vi "Card Inserted.vi"(8 "error in (no error)":errorcluster, 11 "ATM Controller in":refnum<class "ATM Controller.lvclass">) -> (0 "error out":errorcluster, 3 "ATM Controller out":refnum<class "ATM Controller.lvclass">)   [LabVIEW 2020, in "ATM Controller.lvclass"]
uses:
  ATM Controller.lvclass
  State.ctl
  ATM Controller.lvclass/ATM Controller.ctl
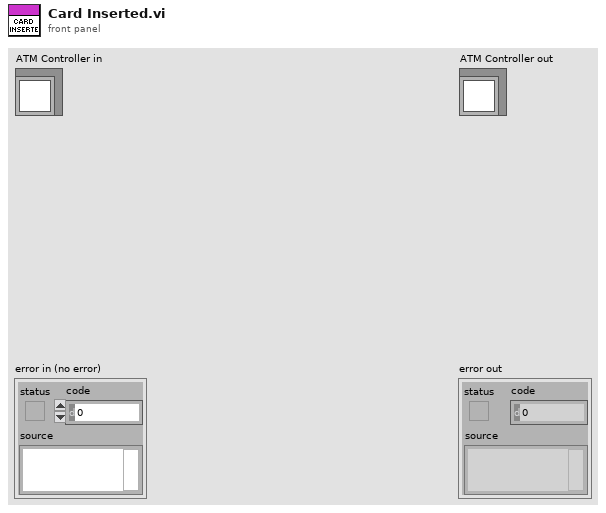
[diagram p1: front panel]
types:
  T1 = typedef "ATM Controller.lvclass/State.ctl" = enum16{"Start", "Card Inserted", "Verification Failed", "Verification Succeeded", "Depositing", "Depositing Completed", "Withdrawing", "Withdraw Completed", "Withdraw Failed", "Balance Inquiry", "Terminate"}
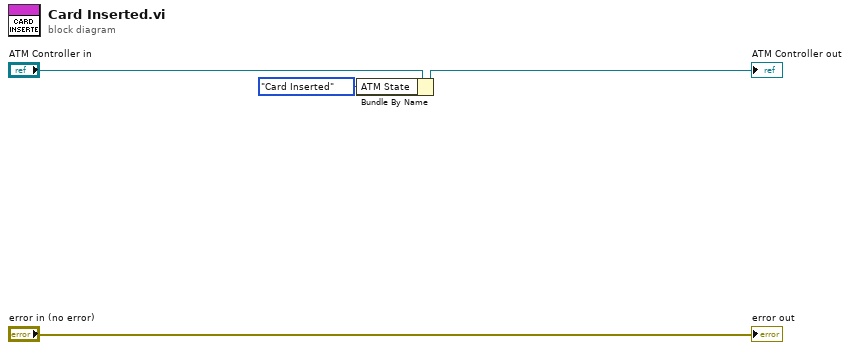
[diagram p0: block diagram]
diagram:
  n1 = Bundle By Name(cluster="ATM Controller in", "ATM State"=State."Card Inserted") -> (→"ATM Controller out":refnum<class "ATM Controller.lvclass">)
  "error out" <- "error in (no error)"
